vi "Receive Message.vi"(6 "priority":i32, 10 "ActorCountsMessageCycles in":refnum<class "ActorCountsMessageCycles.lvclass">, 11 "Message in":refnum<class "Message.lvclass">) -> (0 "error out":errorcluster, 2 "Actor out":refnum<class "Actor.lvclass">)   [LabVIEW 2017, in "ActorCountsMessageCycles.lvclass"]
doc: "This VI should be overriden ONLY if you are creating a proxy actor for remote transmission. If you are, override this VI to transmit the received message to a new destination, maintaining the given priority."
uses:
  ActorCountsMessageCycles.lvclass
  <vilib>/ActorFramework/Message/Message.lvclass
  <vilib>/ActorFramework/Actor/Actor.lvclass
  Source/MessageCycle/MessageCycle.lvclass
  ActorCountsMessageCycles.lvclass/ActorCountsMessageCycles.ctl
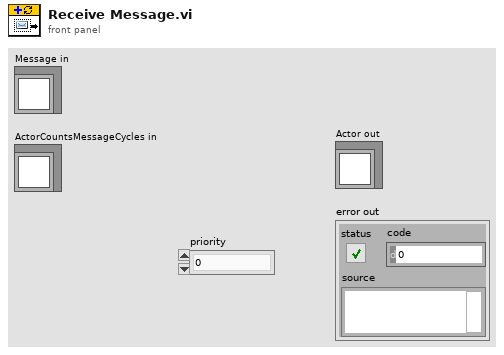
[diagram p1: front panel]
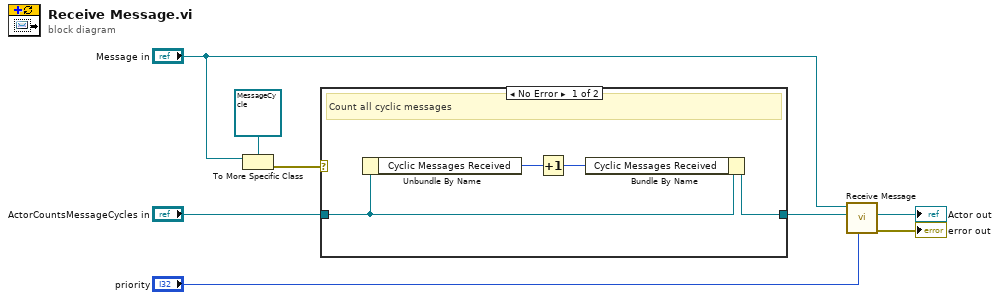
[diagram p0: block diagram]
diagram:
  n1 = To More Specific Class(target class=refnum<class "MessageCycle.lvclass"> refnum ("CyclicMessage.lvclass"), reference="Message in") -> (error out=w1:errorcluster)  [unwired: 1 in, 1 out]
  n2 = case shown="No Error" w1 {
    tunnel: [w12 w13] -> w3
    tunnel: "ActorCountsMessageCycles in" -> [w11 w13]
    frame No Error {
      # "Count all cyclic messages"
      n3 = Unbundle By Name(w11) -> ("Cyclic Messages Received"=w10:u32)
      n4 = Increment(x=w10) -> (x+1=w9:u32)
      n5 = Bundle By Name(cluster=w11, "Cyclic Messages Received"=w9) -> (w12:refnum<class "ActorCountsMessageCycles.lvclass">)
    }
    frame Error {
      # "Not a cyclic message"
    }
  }
  n6 = call-parent "Receive Message.vi"("priority"="priority", "Actor in"=w3, "Message in"="Message in") -> ("error out"=→"error out":errorcluster, "Actor out"=→"Actor out":refnum<class "Actor.lvclass">)  [unwired: 7 in]
